vi "Move Custom Step.vi"(8 "error in (no error)":errorcluster, 10 "Step (mm)":dbl, 11 "Stage Controller in":refnum<class "Stage Controller.lvclass">) -> (0 "error out":errorcluster, 3 "Stage Controller out":refnum<class "Stage Controller.lvclass">)   [LabVIEW 2018, in "Stage Controller.lvlib" / "Stage Controller.lvclass"]
uses:
  Stage Controller.lvclass
  Stage Controller.lvclass/Stage Controller.ctl
  <instrlib>/ASI TG-1000/Public/Utility/Axis Name.ctl
  Ti2/ti2lv/ti2lv.lvlib
  <instrlib>/ASI TG-1000/ASI TG-1000.lvlib
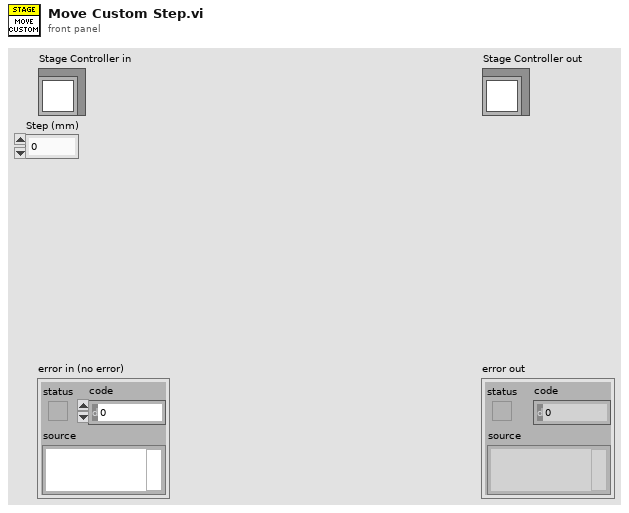
[diagram p1: front panel]
types:
  T1 = enum16{"Disabled", "ESP301", "Ti2", "Ludl", "ASI"}
  T2 = typedef "ASI TG-1000.lvlib/Axis Name.ctl" = enum8{"undefined", "A", "B", "C", "D", "E", "F", "G", "H", "I", "J", "K", "L", "M", "N", "O", "P", "Q", "R", "S", "T", "U", "V", "W", "X", "Y", "Z"}
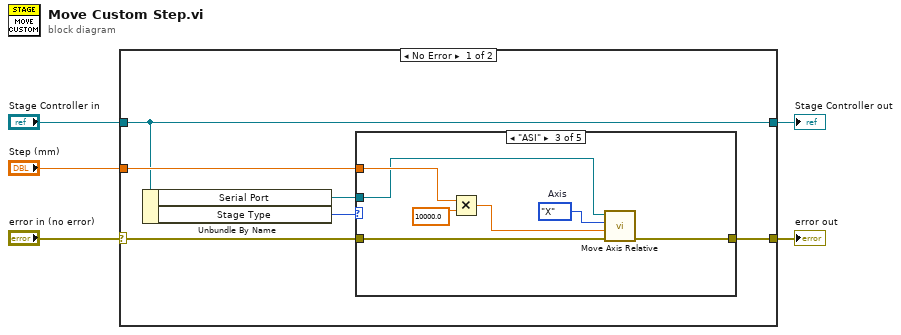
[diagram p0: block diagram]
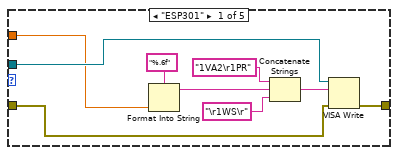
[diagram p2: hidden frame]
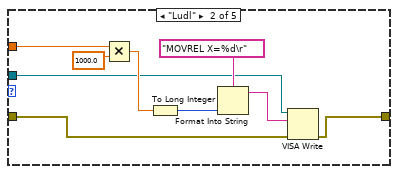
[diagram p3: hidden frame]
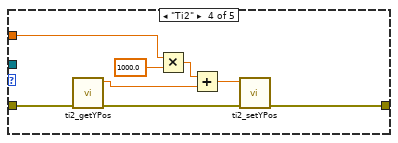
[diagram p4: hidden frame]
diagram:
  n1 = case shown="No Error" "error in (no error)" {
    selector: "error in (no error)" -> [w9 w47]
    tunnel: [w10 w47] -> w4
    tunnel: [w8 w46] -> w2
    tunnel: "Stage Controller in" -> [w8 w46]
    tunnel: "Step (mm)" -> [w11 _]
    frame No Error {
      n2 = Unbundle By Name(w8) -> ("Serial Port"=w7:refnum<visa-resource-name>, "Stage Type"=w6:T1)
      n3 = case shown="\"ASI\"" w6 {
        tunnel: w11 -> [w12 w24 w31 w42 _]
        tunnel: [w14 w22 w33 w41 w45] -> w10
        tunnel: w9 -> [w13 w21 w32 w40 w45]
        tunnel: w7 -> [w15 w23 w30 _ _]
        frame "ESP301" {
          n4 = Format Into String(format string="%.6f", w12) -> (resulting string=w19:string)  [unwired: 2 in, 1 out]
          n5 = Concatenate Strings("1VA2\r1PR" ("write buffer"), w19, "\r1WS\r" ("write buffer")) -> (w20:string)
          n6 = VISA Write(VISA resource name=w15, write buffer=w20, error in (no error)=w13) -> (error out=w14:errorcluster)  [unwired: 2 out]
        }
        frame "Ludl" {
          n7 = Multiply(x=w24, y=1000.0) -> (x*y=w25:dbl)
          n8 = To Long Integer(number=w25) -> (32bit integer=w26:i32)
          n9 = Format Into String(format string="MOVREL X=%d\r", w26) -> (resulting string=w28:string)  [unwired: 2 in, 1 out]
          n10 = VISA Write(VISA resource name=w23, write buffer=w28, error in (no error)=w21) -> (error out=w22:errorcluster)  [unwired: 2 out]
        }
        frame "ASI" {
          w36 = Axis_Name."X"  # Axis
          n11 = Multiply(x=w31, y=10000.0) -> (x*y=w35:dbl)
          n12 = call <instrlib>:"Move Axis Relative.vi"("error in (no error)"=w32, "Relative Position [internal units]"=w35, "Axis"=w36, "VISA in"=w30) -> ("error out"=w33:errorcluster)  [unwired: 5 in, 1 out]
        }
        frame "Ti2" {
          n13 = call "ti2_getYPos.vi"("error in (no error)"=w40) -> ("error out"=w39:errorcluster, "y Position (um)"=w37:dbl)  [unwired: 9 in]
          n14 = Multiply(x=w42, y=1000.0) -> (x*y=w44:dbl)
          n15 = Add(x=w44, y=w37) -> (x+y=w38:dbl)
          n16 = call "ti2_setYPos.vi"("error in (no error)"=w39, "y Position (um)"=w38) -> ("error out"=w41:errorcluster)  [unwired: 9 in]
        }
        frame "Disabled", Default {
        }
      }
    }
    frame Error {
    }
  }
  "error out" <- w4
  "Stage Controller out" <- w2
